vi "B7_65_StandartRangeSelect (SubVI).vi"(1 "Control Point":dbl, 2 "RangeDigit":dbl[](array[numeric]), 4 "RangeCommand":string[](array[string])) -> (0 "R/O":string)   [LabVIEW 2018]
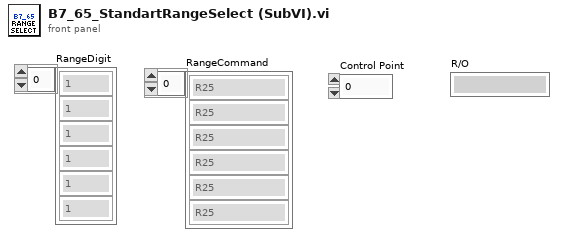
[diagram p1: front panel]
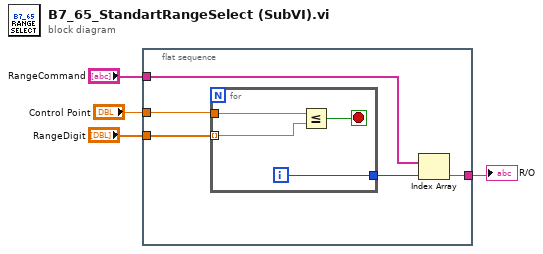
[diagram p0: block diagram]
diagram:
  n1 = flat-sequence {
    tunnel: "Control Point" -> [w9]
    tunnel: "RangeDigit" -> [w8]
    tunnel: "RangeCommand" -> [w7]
    tunnel: [w6] -> w1
    frame #0 {
      n2 = for {
        tunnel: w8 -> [w11] mode=indexing
        tunnel: w9 -> [w12]
        tunnel: [w13] -> w5
        i -> [w13]
        stop <- w10 stop-if-true
        n3 = Less Or Equal?(x=w12, y=w11) -> (x <= y?=w10:bool)
      }
      n4 = Index Array(array=w7, index=w5) -> (element=w6:string)
    }
  }
  "R/O" <- w1
